vi "SCRIPT_EXISTS.vi"(0 "TCP session in":refnum<k5>, 7 "SHA1s":string[](array[string]), 11 "error in":errorcluster) -> (4 "TCP session out":refnum<k5>, 6 "Data":T1, 8 "string data":string[](array[string]), 15 "error out":errorcluster)   [LabVIEW 2023]
uses:
  SubVIs/Controls/redis-data.ctl
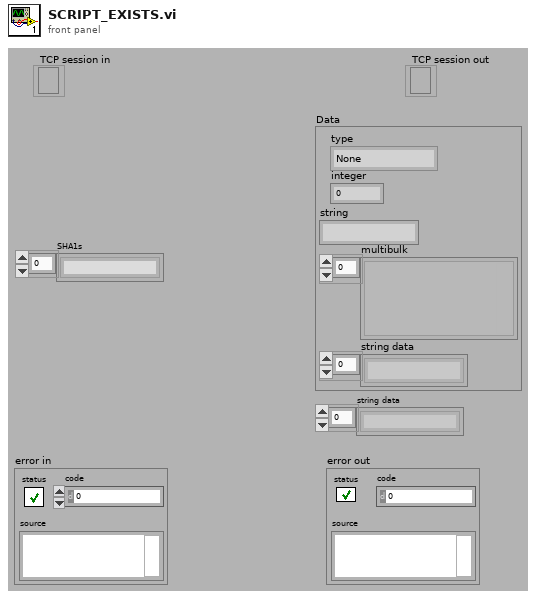
[diagram p1: front panel]
types:
  T1 = typedef "redis-data.ctl" = cluster{"type":enum16{"None", "Error", "Status", "Nil", "Integer", "String", "Multibulk"}, "integer":i64, "string":string, "multibulk":variant[], "string data":string[]}
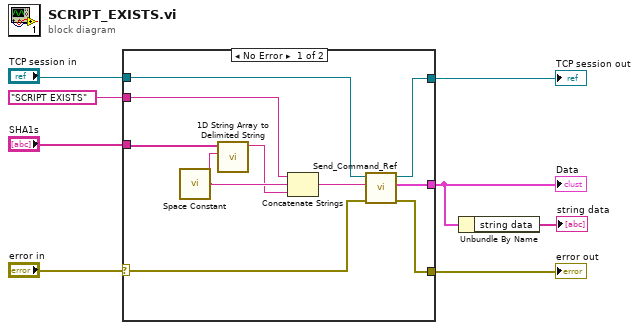
[diagram p0: block diagram]
diagram:
  n1 = case shown="No Error" "error in" {
    selector: "error in" -> [w18 w20]
    tunnel: "SCRIPT EXISTS" -> [w12 _]
    tunnel: "TCP session in" -> [w15 w19]
    tunnel: [w17 w20] -> w6
    tunnel: [w16 _] -> w1
    tunnel: [w14 w19] -> w4
    tunnel: "SHA1s" -> [w11 _]
    frame No Error {
      n2 = call <vilib>:"Space Constant.vi"() -> ("String"=w10:string)
      n3 = call <vilib>:"1D String Array to Delimited String.vi"("delimiter"=w10, "string array"=w11) -> ("delimited string"=w9:string)  [unwired: 9 in]
      n4 = Concatenate Strings(w12, w10, w9) -> (w13:string)
      n5 = call "Send_Command_Ref.vi"("error in"=w18, "command"=w13, "TCP session in"=w15) -> ("error out"=w17:errorcluster, "Data"=w16:T1, "TCP session out"=w14:refnum<k5>)  [unwired: 6 in]
    }
    frame Error {
    }
  }
  "error out" <- w6
  "TCP session out" <- w4
  "Data" <- w1
  n6 = Unbundle By Name(w1) -> ("string data"=→"string data":string[])
